vi "SM_Template.vi"() -> ()   [LabVIEW 2013]
panel:
  in  "AUTO":bool
  in  "CALCU":bool
  in  "TYPE":bool
  in  "Call;":bool
  in  "Write":bool
  in  "クラスタ":cluster{"LED":bool, "Value":i32}
  in  "EXIT":bool
  out "l":i32
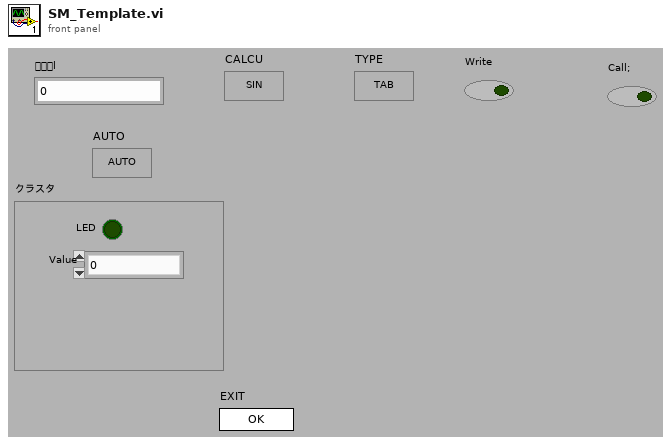
[diagram p1: front panel]
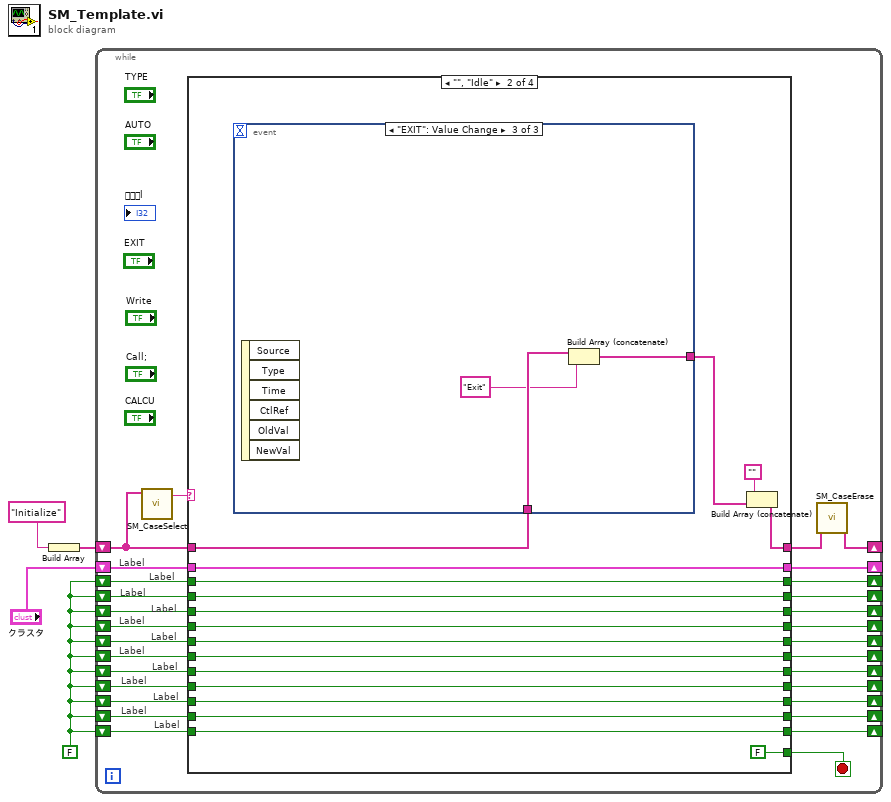
[diagram p0: block diagram]
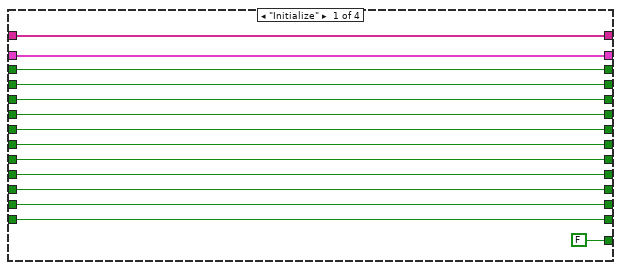
[diagram p2: hidden frame]
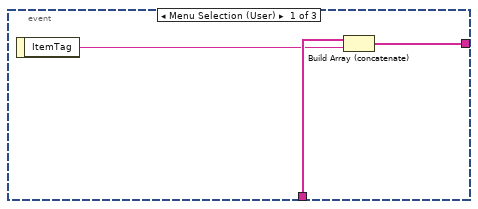
[diagram p3: hidden frame]
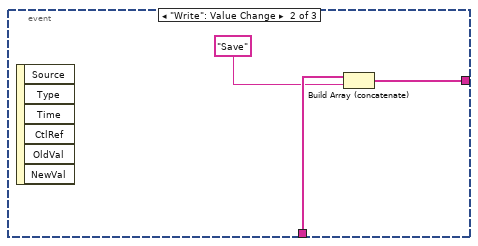
[diagram p4: hidden frame]
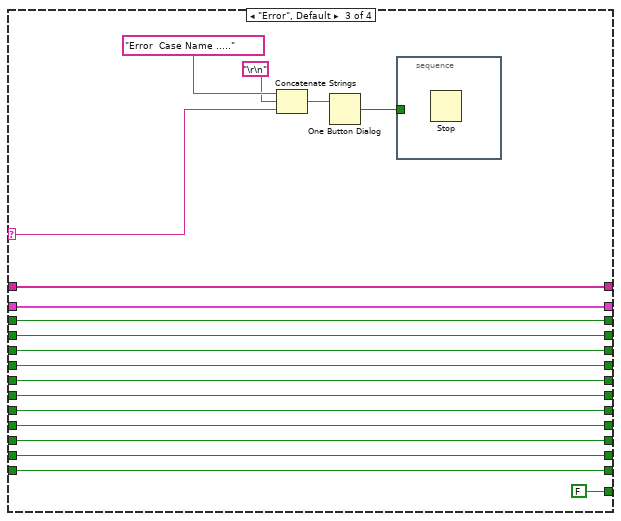
[diagram p5: hidden frame]
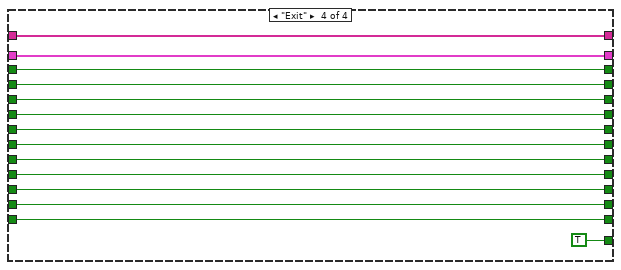
[diagram p6: hidden frame]
diagram:
  w4 = FALSE
  n1 = Build Array("Initialize") -> (w2:string[])
  n2 = while {
    shift-right: [w16] -> _
    shift-left: w4 -> [w17]
    shift-right: [w18] -> _
    shift-left: w4 -> [w19]
    shift-right: [w20] -> _
    shift-left: w4 -> [w21]
    shift-right: [w22] -> _
    shift-left: w4 -> [w23]
    shift-right: [w24] -> _
    shift-left: w4 -> [w25]
    shift-right: [w26] -> _
    shift-left: w4 -> [w27]
    shift-right: [w28] -> _
    shift-left: "クラスタ" -> [w29]
    shift-right: [w14] -> _
    shift-left: w4 -> [w15]
    shift-right: [w32] -> _
    shift-left: w4 -> [w33]
    shift-right: [w11] -> _
    shift-left: w2 -> [w30]
    shift-right: [w9] -> _
    shift-left: w4 -> [w10]
    shift-right: [w7] -> _
    shift-left: w4 -> [w8]
    shift-right: [w6] -> _
    shift-left: w4 -> [w5]
    stop <- w13 stop-if-true
    # "Label"
    # "Label"
    # "Label"
    # "Label"
    # "Label"
    # "Label"
    # "Label"
    # "Label"
    # "Label"
    # "Label"
    # "Label"
    # "Label"
    n3 = call "SM_CaseSelect.vi"("Input"=w30) -> ("Case"=w31:string)  [unwired: 10 out]
    n4 = case shown="\"\", \"Idle\"" w31 {
      selector: w31 -> [_ _ w74 _]
      tunnel: w33 -> [w47 w64 w92 w106]
      tunnel: [w47 w64 w92 w106] -> w32
      tunnel: w30 -> [w46 w51 w91 w105]
      tunnel: [w46 w48 w91 w105] -> w12
      tunnel: w29 -> [w45 w63 w90 w104]
      tunnel: [w45 w63 w90 w104] -> w28
      tunnel: w27 -> [w44 w62 w89 w103]
      tunnel: [w44 w62 w89 w103] -> w26
      tunnel: w25 -> [w43 w61 w88 w102]
      tunnel: [w43 w61 w88 w102] -> w24
      tunnel: w23 -> [w42 w60 w87 w101]
      tunnel: [w42 w60 w87 w101] -> w22
      tunnel: w21 -> [w41 w59 w86 w100]
      tunnel: [w41 w59 w86 w100] -> w20
      tunnel: w19 -> [w40 w58 w85 w99]
      tunnel: [w40 w58 w85 w99] -> w18
      tunnel: w17 -> [w39 w57 w84 w98]
      tunnel: [w39 w57 w84 w98] -> w16
      tunnel: w15 -> [w38 w56 w83 w97]
      tunnel: [w38 w56 w83 w97] -> w14
      tunnel: [FALSE FALSE FALSE TRUE] -> w13
      tunnel: w10 -> [w34 w52 w79 w93]
      tunnel: [w34 w52 w79 w93] -> w9
      tunnel: w8 -> [w36 w54 w81 w95]
      tunnel: [w36 w54 w81 w95] -> w7
      tunnel: [w35 w53 w80 w94] -> w6
      tunnel: w5 -> [w35 w53 w80 w94]
      frame "Initialize" {
      }
      frame "", "Idle" {
        n5 = event shown="[2] \"EXIT\": lÏX" {
          selector: _ -> [_ _ _]
          dyn-events: _ -> [_ _ _]
          timeout: _ -> [_ _ _]
          tunnel: w51 -> [w67 w70 w73]
          tunnel: [w65 w69 w72] -> w49
          event Menu Selection (User) {
            n6 = event-data() -> ("ItemTag"=w66:string)  [unwired: 1 out]
            n7 = Build Array (concatenate)(w67, w66) -> (w65:string[])
          }
          event "Write": Value Change {
            n8 = event-data() -> ()  [unwired: 7 out]
            n9 = Build Array (concatenate)(w70, "Save") -> (w69:string[])
          }
          event "EXIT": Value Change {
            n10 = event-data() -> ()  [unwired: 7 out]
            n11 = Build Array (concatenate)(w73, "Exit") -> (w72:string[])
          }
        }
        n12 = Build Array (concatenate)("", w49) -> (w48:string[])
      }
      frame "Error", Default {
        n13 = Concatenate Strings("Error  Case Name .....", "\r\n", w74) -> (w76:string)
        n14 = One Button Dialog(message=w76) -> (true=w75:bool)  [unwired: 1 out]
        n15 = stacked-sequence {
          tunnel: w75 -> [_]
          frame #0 {
            n16 = Stop() -> ()  [unwired: 1 out]
          }
        }
      }
      frame "Exit" {
      }
    }
    n17 = call "SM_CaseErase.vi"("Input"=w12) -> ("Output"=w11:string[])  [unwired: 10 out]
  }
